vi "FromRepo.vi"(8 "error in":errorcluster, 9 "from repo cluster":T2, 10 "repository in":refnum<class "NISE_CEF_Repository.lvclass">, 11 "group in":refnum<class "device.lvclass">) -> (0 "error out":errorcluster, 2 "repository out":refnum<class "NISE_CEF_Repository.lvclass">, 3 "root":T1)   [LabVIEW 2013, in "device.lvclass"]
uses:
  device.lvclass
  <vilib>/NI/Configuration Framework/Repository/NISE_CEF_Repository.lvclass
  <vilib>/NI/Configuration Framework/Node/FromRepoCluster.ctl
  <vilib>/NI/Configuration Framework/Node/NodeRef.ctl
  <vilib>/NI/Configuration Framework/Node/NISE_CEF_Node.lvclass
  database file/database file.lvclass
  database file/database file.lvclass/database file.ctl
  device.lvclass/device.ctl
  database file/Read frames.vi
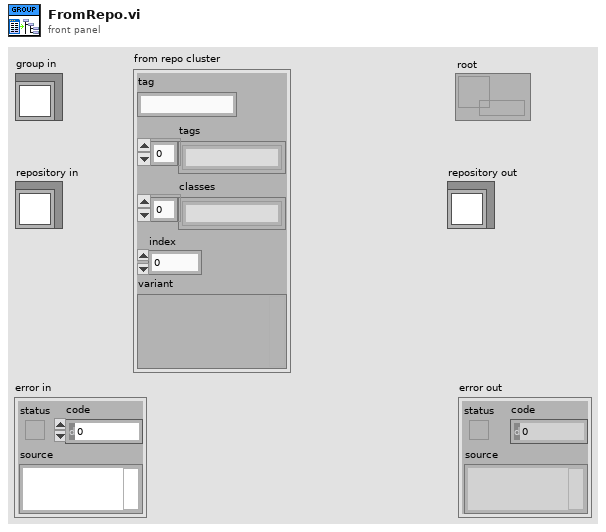
[diagram p1: front panel]
types:
  T1 = typedef "NISE_CEF_Node.lvclass/NodeRef.ctl" = refnum<data-value>
  T2 = typedef "NISE_CEF_Node.lvclass/FromRepoCluster.ctl" = cluster{"tag":string, "tags":string[], "classes":string[], "index":i32, "variant":variant}
  T3 = typedef "J1939.lvlib/J1939 db frame.ctl" = cluster{"name":string, "Priority":u8, "PGN":u32, "Reserved Bit":u8, "Data page":u8, "PDU Format":u8, "PDU Specific":u8, "Source Address":u8, "PayldLen":u32, "signals":T4[], "Comment":string, "can timing type":u32, "transmit time":dbl, "direction":u16}
  T4 = typedef "J1939.lvlib/J1939 db signal.ctl" = cluster{"NameShort":string, "SPN":i32, "StartBit":u32, "NumBits":u32, "DataType":u32, "ByteOrdr":u32, "ScaleFac":dbl, "ScaleOff":dbl, "Max":dbl, "Min":dbl, "Default":dbl, "Unit":string, "Comment":string}
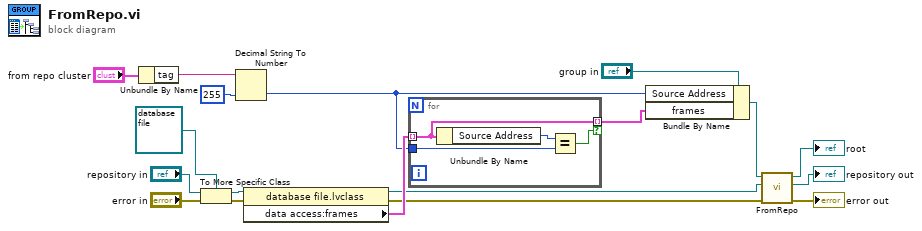
[diagram p0: block diagram]
diagram:
  n1 = Unbundle By Name("from repo cluster") -> ("tag"=w6:string)
  n2 = To More Specific Class(target class=refnum<class "database file.lvclass"> refnum ("cRIO repo.lvclass"), reference="repository in", error in="error in") -> (specific class reference=w16:refnum<class "database file.lvclass">, error out=w14:errorcluster)
  n3 = Decimal String To Number(string=w6, default (0L)=u8 255 ("default (0 I32)")) -> (number=w3:u8)  [unwired: 1 in, 1 out]
  n4 = property class="database file.lvclass"(reference=w16, error in=w14) -> (reference out=w8:refnum<class "database file.lvclass">, error out=w1:errorcluster, "data access:frames"=w15:T3[])
  n5 = for {
    tunnel: w15 -> [w20] mode=indexing
    tunnel: w3 -> [w21]
    tunnel: [w20] -> w2 mode=indexing if=w19
    n6 = Unbundle By Name(w20) -> ("Source Address"=w22:u8)
    n7 = Equal?(x=w22, y=w21) -> (x = y?=w19:bool)
  }
  n8 = Bundle By Name(cluster="group in", "Source Address"=w3, "frames"=w2) -> (w4:refnum<class "device.lvclass">)
  n9 = call-parent "FromRepo.vi"("error in"=w1, "repository in"=w8, "node in"=w4) -> ("error out"=→"error out":errorcluster, "repository out"=→"repository out":refnum<class "NISE_CEF_Repository.lvclass">, "node"=→"root":T1)  [unwired: 6 in]
